vi "SR620_single_read_data.vi"(0 "SR620_No.1_Port":refnum<visa-resource-name>="GPIB0::19::INSTR", 1 "Channel (1: A)":i32(ring)=1 items=["Ext Input", "A", "B"], 2 "SR620_No.1 (2: REF)":i32(ring) items=["A", "B", "REF", "A / B"], 3 "Meas. Mode (0: Time)":i32(ring) items=["Time", "Width", "Rise / Fall Time", "Frequency", "Period", "Phase", "Count"], 4 "Arming Mode\n (0: +/-time)":i32(ring)=1 items=["+/-time", "+time", "1 period", "0.01s gate", "0.1s gate", "1.0s gate", "ext trig +/- time", "ext trig +time", "ext gate/+ time/hldf", "ext triggered 1 period", "ext triggered .01s gate", "ext triggered 0.1s gate", "ext triggered 1.0s gate"], 5 "Gate Time (Auto)":dbl(ring) items=["Auto"=0.0, "1E-6"=1e-06, "2E-6"=2e-06, "5E-6"=5e-06, "1E-5"=1e-05, "2E-5"=2e-05, "5E-5"=5e-05, "1E-4"=0.0001, "2E-4"=0.0002, "5E-4"=0.0005, "1E-3"=0.001, "2E-3"=0.002, "5E-3"=0.005, ".01"=0.01, ".02"=0.02, ".05"=0.05, ".1"=0.1, ".2"=0.2, ".5"=0.5, "1"=1.0, "2"=2.0, "5"=5.0, "10"=10.0, "20"=20.0, "50"=50.0, "100"=100.0, "200"=200.0, "500"=500.0], 6 "Sample Size (1)":u32(ring)=1 items=["1"=1, "2"=2, "5"=5, "10"=10, "20"=20, "50"=50, "100"=100, "200"=200, "500"=500, "1000"=1000, "2000"=2000, "5000"=5000, "10000"=10000, "20000"=20000, "50000"=50000, "100000"=100000, "200000"=200000, "500000"=500000, "1000000"=1000000], 7 "SR620_No.1 error in\n (no error)":errorcluster, 8 "Input Termination_ (0: 50 Ohms)":i32(ring) items=["50 Ohms", "1 Mohm", "UHF Prescalers"], 9 "Timeout (25000 ms)":u32=1000 step=1000, 10 "Coupling (F: DC)":bool, 11 "Ref Out (1: TTL)":i32(ring)=1 items=["ECL", "TTL"], 12 "Auto Trigger Level (True)":bool, 14 "Trigger Level (0.00 V)":dbl=1.0, 16 "Trigger Slope (T: Positive)":bool=TRUE) -> (20 "SR620_No.1":refnum<visa-resource-name>="GPIB0::19::INSTR", 27 "SR620_No1\nerror out":errorcluster)   [LabVIEW 2014]
doc: "Provides an example of how to use the SR620 subVIs programmatically."
uses:
  <vilib>/Utility/file.llb/Write To Spreadsheet File (DBL).vi
panel:
  out "SR620_Delta_T":dbl format="%.12f"
  in  "delimiter (\\n)":string="\n" caption="数据分隔符(\\n)"
  in  "文件路径: single":path=path "C:/Users/Administrator/Desktop/PID_Discipline_WithoutSystem_X72_Single/single_read_data.txt"
  out "本地测量钟差":dbl[](graph)=[7593300.0, 241.375901, 241.375903, 241.375876, 241.375868, 241.375803, 241.375857, 241.375887, 241.375852, 241.37583800000002, 241.37586299999998]
  out "总计数值":i32
  in  "控制开关":bool
  # "SR620数据测量显示"
  # "Delta_T"
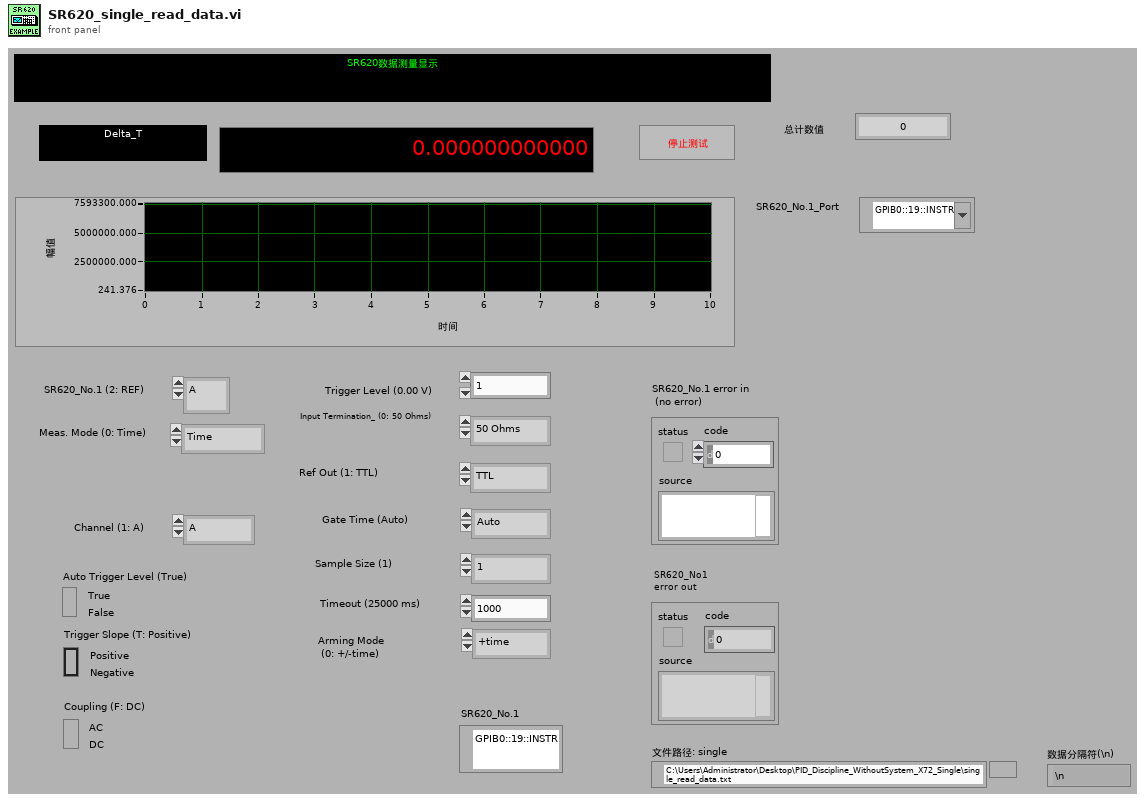
[diagram p1: front panel]
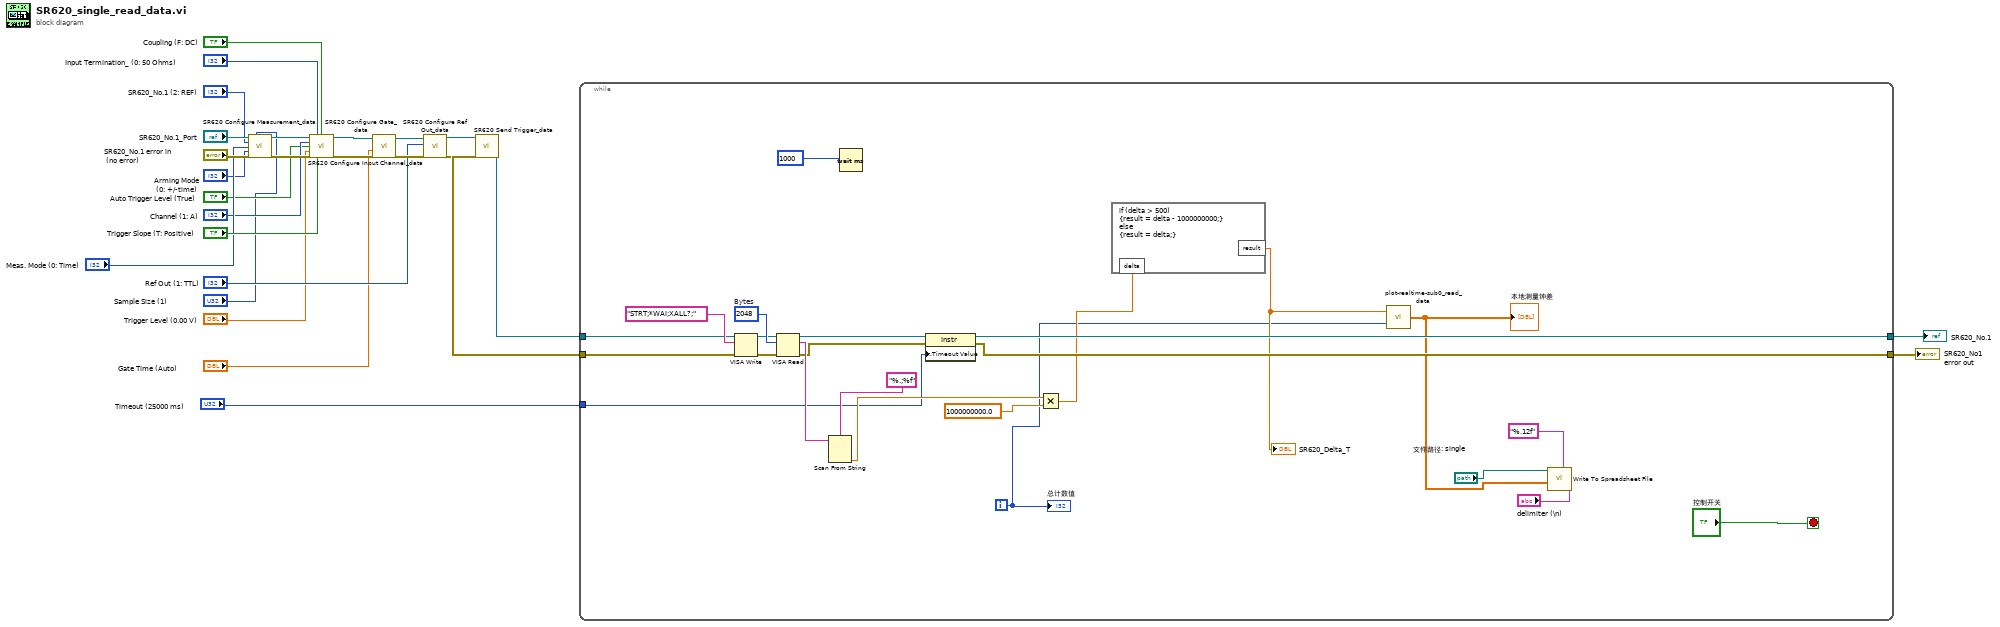
[diagram p0: block diagram]
diagram:
  n1 = call "SR620 Configure Measurement_data.vi"("VISA session"="SR620_No.1_Port", "Sample Size (1)"="Sample Size (1)", "Source (2: REF)"="SR620_No.1 (2: REF)", "Measurement Mode (0: Time)"="Meas. Mode (0: Time)", "Arming Mode (0: +/-time)"="Arming Mode\n (0: +/-time)", "error in (no error)"="SR620_No.1 error in\n (no error)") -> ("dup VISA session"=w19:refnum<visa-resource-name>, "error out"=w17:errorcluster)  [unwired: 8 in]
  n2 = call "SR620 Configure Input Channel_data.vi"("VISA session"=w19, "Input Termination (0: 50 Ohms)"="Input Termination_ (0: 50 Ohms)", "Coupling (F: DC)"="Coupling (F: DC)", "Channel (1: A)"="Channel (1: A)", "Auto Trigger Level (True)"="Auto Trigger Level (True)", "Trigger Level (0.00 V)"="Trigger Level (0.00 V)", "error in (no error)"=w17, "Trigger Slope (T: Positive)"="Trigger Slope (T: Positive)") -> ("dup VISA session"=w18:refnum<visa-resource-name>, "error out"=w16:errorcluster)  [unwired: 6 in]
  n3 = call "SR620 Configure Gate_data.vi"("error in (no error)"=w16, "Gate Time (Auto)"="Gate Time (Auto)", "VISA session"=w18) -> ("error out"=w21:errorcluster, "dup VISA session"=w20:refnum<visa-resource-name>)  [unwired: 5 in]
  n4 = call "SR620 Configure Ref Out_data.vi"("error in (no error)"=w21, "Amplitude: Ref Output (1: TTL)"="Ref Out (1: TTL)", "VISA session"=w20) -> ("error out"=w22:errorcluster, "dup VISA session"=w23:refnum<visa-resource-name>)  [unwired: 3 in]
  n5 = call "SR620 Send Trigger_data.vi"("VISA session"=w23, "error in (no error)"=w22) -> ("dup VISA session"=w26:refnum<visa-resource-name>, "error out"=w25:errorcluster)  [unwired: 12 in]
  n6 = while {
    tunnel: w26 -> [w45]
    tunnel: w25 -> [w44]
    tunnel: [w43] -> w14
    tunnel: [w42] -> w13
    tunnel: "Timeout (25000 ms)" -> [w38]
    i -> [w30]
    stop <- "控制开关" stop-if-true
    w51 = u32 2048  # Bytes
    n7 = VISA Write(VISA resource name=w45, write buffer="STRT;*WAI;XALL?;" ("write buffer (\"\")"), error in (no error)=w44) -> (VISA resource name out=w29:refnum<visa-resource-name>, error out=w28:errorcluster)  [unwired: 1 out]
    n8 = VISA Read(VISA resource name=w29, byte count=w51, error in (no error)=w28) -> (VISA resource name out=w47:refnum<visa-resource-name>, read buffer=w48:string, error out=w46:errorcluster)  [unwired: 1 out]
    n9 = Scan From String(format string="%.;%f", input string=w48) -> (output 1=w40:dbl)  [unwired: 3 in, 3 out]
    n10 = Wait (ms)(milliseconds to wait=1000) -> ()  [unwired: 1 out]
    n11 = property class="Instr"(reference=w47, error in=w46, "General Settings:Timeout Value"=w38) -> (reference out=w43:refnum<visa-resource-name>, error out=w42:errorcluster)
    n12 = Multiply(x=w40, y=1000000000.0) -> (x*y=w32:dbl)
    n13 = formula code="if (delta > 500)\n{result = delta - 1000000000;}\nelse\n{result = delta;}"("delta"=w32) -> ("result"=w31:dbl)
    "SR620_Delta_T" <- w31
    n14 = call "plot-realtime-sub0_read_data.vi"("索引"=w30, "x"=w31) -> ("数组"=w33:dbl[])
    "本地测量钟差" <- w33
    n15 = call-poly <vilib>:"Write To Spreadsheet File.vi"("delimiter (\\t)"="delimiter (\\n)", "format (%.3f)"="%.12f", "1D data"=w33, "file path (dialog if empty)"="文件路径: single") -> ()  [unwired: 4 in, 1 out]
    "总计数值" <- w30
  }
  "SR620_No.1" <- w14
  "SR620_No1\nerror out" <- w13
